vi "BeepGen2.vi"(9 "Wait time before beep (s)":dbl, 11 "Time b/w Beeps (s)":dbl=3.0) -> (0 "x/y":dbl, 2 "In Range?":bool, 3 "Numeric out":dbl)   [LabVIEW 2019]
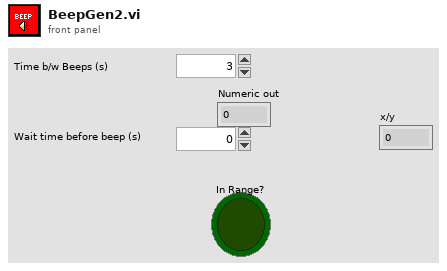
[diagram p1: front panel]
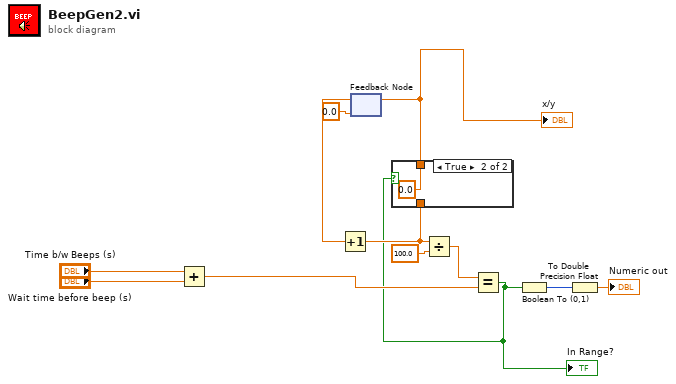
[diagram p0: block diagram]
diagram:
  n1 = Add(x="Time b/w Beeps (s)", y="Wait time before beep (s)") -> (x+y=w2:dbl)
  n2 = feedback #1(0.0) -> (w9:dbl)
  n3 = Increment(x=w9) -> (x+1=w5:dbl)
  n4 = Divide(x=w5, y=100.0) -> (x/y=w3:dbl)
  n5 = Equal?(x=w3, y=w2) -> (x = y?=w1:bool)
  "In Range?" <- w1
  n6 = case shown="True" w1 {
    tunnel: [w13 0.0] -> w4
    tunnel: w5 -> [w13 _]
    frame False {
    }
    frame True {
    }
  }
  "x/y" <- w4
  n7 = feedback-in #1(w4) -> ()
  n8 = Boolean To (0,1)(Boolean=w1) -> (0, 1=w11:i16)
  n9 = To Double Precision Float(number=w11) -> (double precision float=→"Numeric out":dbl)
